vi "Calculate Loss (Power Gain Definition).vi"(5 "Termination":cdb[](array[numeric]), 6 "error in (no error)":errorcluster, 9 "S-parameters":cdb[][](array[numeric])) -> (0 "error out":errorcluster, 3 "Loss":dbl[](array[numeric]))   [LabVIEW 2023, in "NI_HFNetworkAnalysis.lvlib"]
doc: "Calculates the mismatch loss of a 2-port network at different frequencies when it is terminated by the specified termination.\n\nMismatch loss is calculated using <b>power gain definition</b>.\n\nThe network is defined by 2-port S-parameters <b>(S11,S12,S21,S22)</b> at different frequencies and the termination is described by its reflection factor at those frequencies.\n\n<b>Known Limitations</b>\nOnly 2-port networks are supported."
uses:
  NI_HFNetworkAnalysis.lvlib
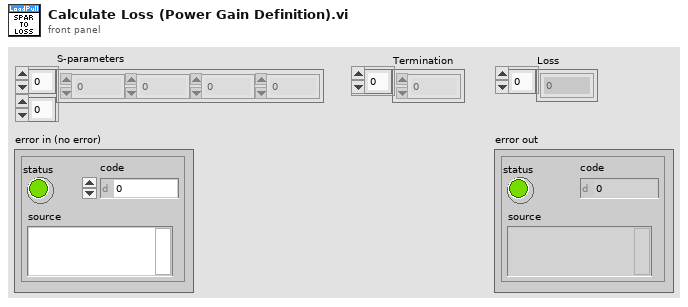
[diagram p1: front panel]
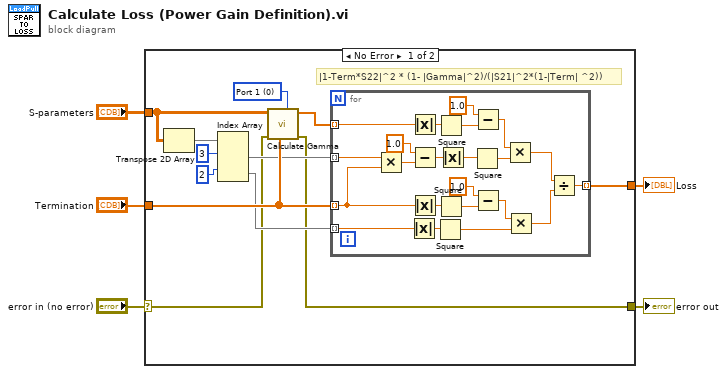
[diagram p0: block diagram]
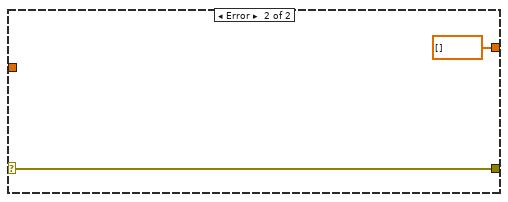
[diagram p2: hidden frame]
diagram:
  n1 = case shown="No Error" "error in (no error)" {
    selector: "error in (no error)" -> [w8 w41]
    tunnel: [w17 dbl[] []] -> w5
    tunnel: "Termination" -> [w15 _]
    tunnel: "S-parameters" -> [w13 _]
    tunnel: [w7 w41] -> w1
    frame No Error {
      w6 = u16 0 items=["Port 1", "Port 2"] ("Port")
      # "|1-Term*S22|^2 * (1- |Gamma|^2)/(|S21|^2*(1-|Term| ^2))"
      n2 = Transpose 2D Array(2D array=w13) -> (transposed array=w14:cdb[][])
      n3 = Index Array(array=w14, index (row) #1=3 ("index (row)"), index (row) #2=2 ("index (row)")) -> (element #1=w10:cdb[], element #2=w9:cdb[])  [unwired: 2 in]
      n4 = call "Calculate Gamma.vi"("Port (Port 1)"=w6, "Termination"=w15, "error in (no error)"=w8, "2-port S-parameters"=w13) -> ("error out"=w7:errorcluster, "Gamma"=w16:cdb[])  [unwired: 4 in]
      n5 = for {
        tunnel: [w20] -> w17 mode=indexing
        tunnel: w16 -> [w32] mode=indexing
        tunnel: w15 -> [w29] mode=indexing
        tunnel: w10 -> [w19] mode=indexing
        tunnel: w9 -> [w18] mode=indexing
        n6 = Multiply(x=w19, y=w29) -> (x*y=w27:cdb)
        n7 = Absolute Value(x=w18) -> (abs(x)=w36:dbl)
        n8 = Absolute Value(x=w32) -> (abs(x)=w31:dbl)
        n9 = Subtract(x=1.0, y=w27) -> (x-y=w26:cdb)
        n10 = Absolute Value(x=w29) -> (abs(x)=w38:dbl)
        n11 = Square(x=w36) -> (x^2=w35:dbl)
        n12 = Square(x=w31) -> (x^2=w30:dbl)
        n13 = Square(x=w38) -> (x^2=w37:dbl)
        n14 = Absolute Value(x=w26) -> (abs(x)=w25:dbl)
        n15 = Square(x=w25) -> (x^2=w24:dbl)
        n16 = Subtract(x=1.0, y=w30) -> (x-y=w23:dbl)
        n17 = Subtract(x=1.0, y=w37) -> (x-y=w34:dbl)
        n18 = Multiply(x=w23, y=w24) -> (x*y=w22:dbl)
        n19 = Multiply(x=w34, y=w35) -> (x*y=w21:dbl)
        n20 = Divide(x=w22, y=w21) -> (x/y=w20:dbl)
      }
    }
    frame Error {
    }
  }
  "Loss" <- w5
  "error out" <- w1
